vi "4.3.vi"() -> ()   [LabVIEW 2017]
panel:
  out "XY图":cluster{dbl[], dbl[]}(graph)
  # "任务三"
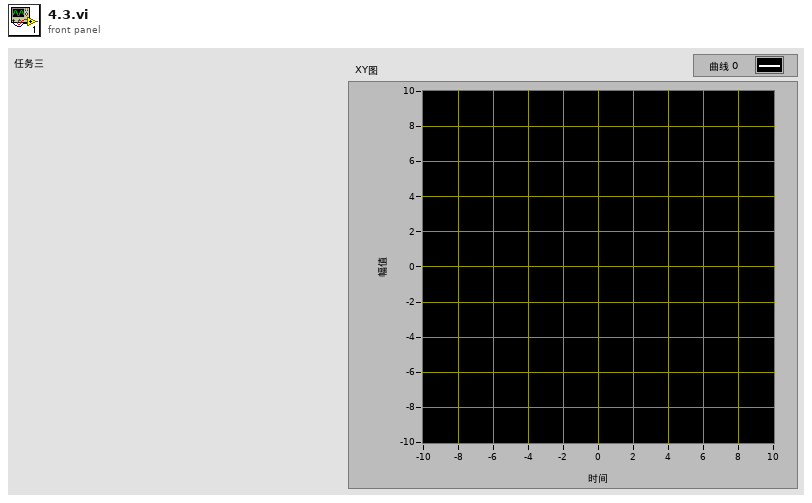
[diagram p1: front panel]
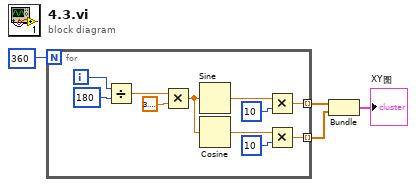
[diagram p0: block diagram]
diagram:
  n1 = for {
    N: 360 -> [_]
    tunnel: [w7] -> w3 mode=indexing
    tunnel: [w5] -> w2 mode=indexing
    i -> [w15]
    n2 = Divide(x=w15, y=180) -> (x/y=w13:dbl)
    n3 = Multiply(x=w13, y=3.141592653589793) -> (x*y=w11:dbl)
    n4 = Sine(x=w11) -> (sin(x)=w8:dbl)
    n5 = Cosine(x=w11) -> (cos(x)=w6:dbl)
    n6 = Multiply(x=w8, y=10) -> (x*y=w7:dbl)
    n7 = Multiply(x=w6, y=10) -> (x*y=w5:dbl)
  }
  n8 = Bundle(w3, w2) -> (→"XY图":cluster{dbl[], dbl[]})  [unwired: 1 in]
